vi "Sum 2D [ox] (DBL).vi"(1 "2D":dbl[][](array[numeric])) -> (0 "1D":dbl[](array[numeric]))   [LabVIEW 2009]
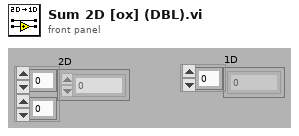
[diagram p1: front panel]
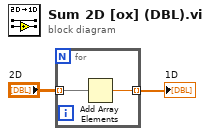
[diagram p0: block diagram]
diagram:
  n1 = for {
    tunnel: "2D" -> [w4] mode=indexing
    tunnel: [w3] -> w1 mode=indexing
    n2 = Add Array Elements(numeric array=w4) -> (sum=w3:dbl)
  }
  "1D" <- w1
